vi "Select Poll List Tags.vi"(8 "error in (no error)":errorcluster, 11 "Node Ptr":T1=18446744073709551615 format="%.0x") -> (0 "error out":errorcluster)   [LabVIEW 2013, in "OPC UA Client System Explorer.lvlib"]
uses:
  OPC UA Client System Explorer.lvlib
  <vilib>/NI Veristand/Custom Device API/Custom Device Item Ref.ctl
  <vilib>/NI Veristand/Custom Device API/Get Item Property (Dependent Node Pointer).vi
  <vilib>/NI Veristand/Custom Device API/Set Item Property (Dependent Node Pointer).vi
  <vilib>/NI Veristand/Custom Device API/Custom Device API.lvlib
  <vilib>/NI Veristand/Custom Device Tools/Custom Device Utility Library/Custom Device Utility Library.lvlib
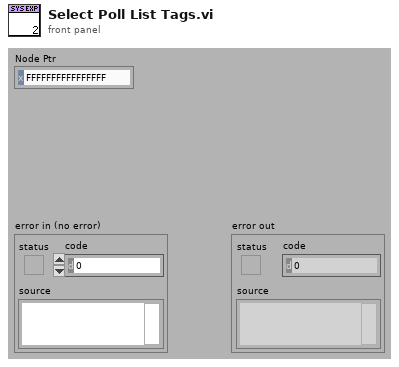
[diagram p1: front panel]
types:
  T1 = typedef "Custom Device API.lvlib/Custom Device Item Ref.ctl" = u64
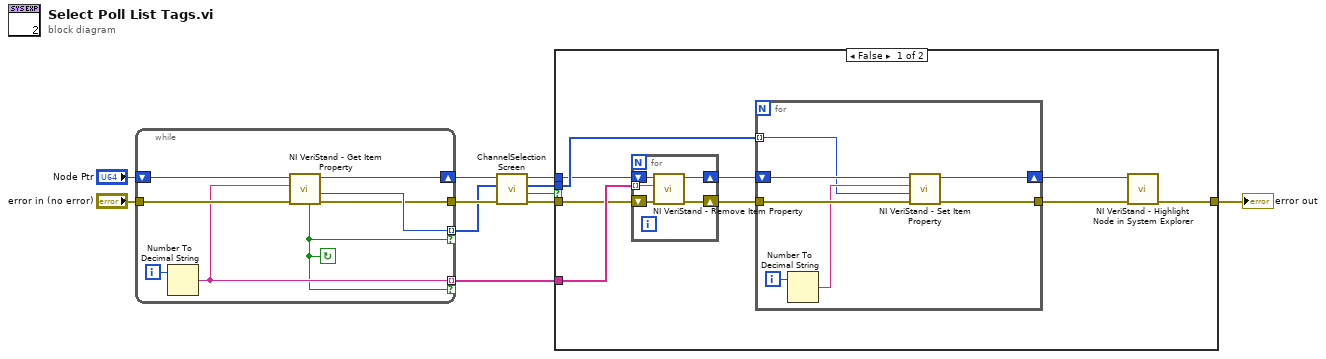
[diagram p0: block diagram]
diagram:
  n1 = while {
    tunnel: "error in (no error)" -> [w18]
    tunnel: [w12] -> w9
    tunnel: [w14] -> w5 mode=indexing if=w13
    shift-right: [w16] -> w8
    shift-left: "Node Ptr" -> [w19]
    tunnel: [w15] -> w4 mode=indexing if=w13
    i -> [w17]
    stop <- w13 continue-if-true
    n2 = Number To Decimal String(number=w17) -> (decimal integer string=w15:string)  [unwired: 1 in]
    n3 = call-poly <vilib>:"NI VeriStand - Get Item Property.vi"("error in (no error)"=w18, "Property Name"=w15, "Item Ref in"=w19) -> ("error out"=w12:errorcluster, "Dependent Node Ref"=w14:T1, "Item Ref out"=w16:T1, "Found"=w13:bool)  [unwired: 5 in]
  }
  n4 = call "ChannelSelectionScreen.vi"("error in"=w9, "Refs"=w5, "Parent Ref"=w8) -> ("error out"=w3:errorcluster, "Cancelled?"=w1:bool, "Refs out"=w6:T1[], "Parent Ref Out"=w2:T1)  [unwired: 5 in]
  n5 = case shown="False" w1 {
    tunnel: [w21 w41] -> w7
    tunnel: w6 -> [w28 _]
    tunnel: w4 -> [w27 _]
    tunnel: w3 -> [w26 w41]
    tunnel: w2 -> [w24 _]
    frame False {
      n6 = for {
        tunnel: w27 -> [w33] mode=indexing
        shift-right: [w31] -> w25
        shift-left: w26 -> [w32]
        shift-right: [w29] -> w23
        shift-left: w24 -> [w30]
        n7 = call <vilib>:"NI VeriStand - Remove Item Property.vi"("error in (no error)"=w32, "Property Name"=w33, "Item Ref in"=w30) -> ("error out"=w31:errorcluster, "Item Ref out"=w29:T1)  [unwired: 6 in, 1 out]
      }
      n8 = for {
        tunnel: w25 -> [w39]
        tunnel: [w38] -> w20
        shift-right: [w35] -> w22
        shift-left: w23 -> [w40]
        tunnel: w28 -> [w34] mode=indexing
        i -> [w37]
        n9 = Number To Decimal String(number=w37) -> (decimal integer string=w36:string)  [unwired: 1 in]
        n10 = call-poly <vilib>:"NI VeriStand - Set Item Property.vi"("error in (no error)"=w39, "Dependent Node Ref"=w34, "Property Name"=w36, "Item Ref in"=w40) -> ("error out"=w38:errorcluster, "Item Ref out"=w35:T1)  [unwired: 5 in, 1 out]
      }
      n11 = call <vilib>:"NI VeriStand - Highlight Node in System Explorer.vi"("error in (no error)"=w20, "Item Ref in"=w22) -> ("error out"=w21:errorcluster)  [unwired: 8 in, 1 out]
    }
    frame True {
    }
  }
  "error out" <- w7
